vi "Get Port.vi"(8 "error in (no error)":errorcluster, 11 "Example Instrument in":refnum<class "Example Instrument.lvclass">) -> (0 "error out":errorcluster, 2 "port":u32, 3 "Example Instrument out":refnum<class "Example Instrument.lvclass">)   [LabVIEW 2016, in "Example Instrument.lvclass"]
uses:
  Example Instrument.lvclass
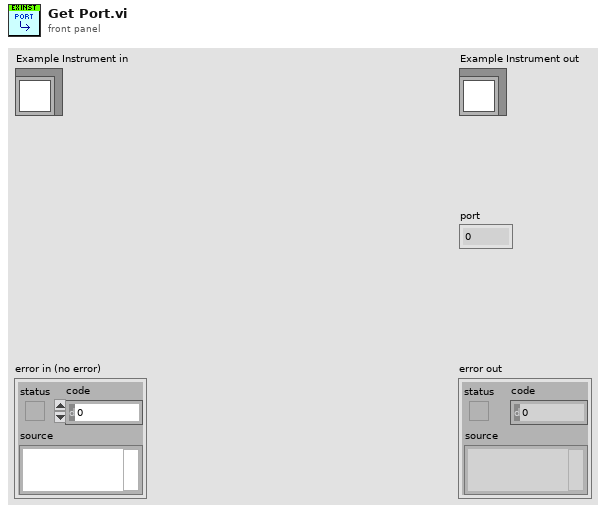
[diagram p1: front panel]
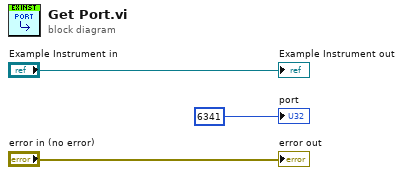
[diagram p0: block diagram]
diagram:
  "error out" <- "error in (no error)"
  "Example Instrument out" <- "Example Instrument in"
  "port" <- u32 6341 ("port")
